vi "Global 1.vi"() -> ()   [LabVIEW 2024]
uses:
  Configuration/Calibration Configuration.ctl
panel:
  in  "Calibration Configuration Out":T1
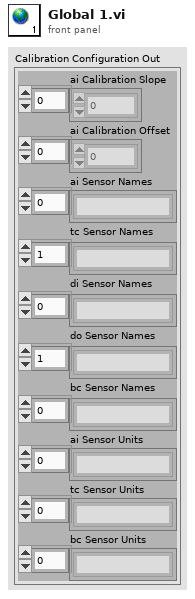
[diagram p1: front panel]
types:
  T1 = typedef "Calibration Configuration.ctl" = cluster{"ai Calibration Slope":dbl[], "ai Calibration Offset":dbl[], "ai Sensor Names ":string[], "tc Sensor Names":string[], "di Sensor Names":string[], "do Sensor Names":string[], "bc Sensor Names":string[], "ai Sensor Units":string[], "tc Sensor Units":string[], "bc Sensor Units":string[]}
diagram:
